vi "Write_CmdMultipleParam.vi"(6 "Command":enum16{"ST"}(ring), 7 "MainParam":i16=-1, 8 "error in (no error)":errorcluster, 9 "Table2":u16[](array[numeric]), 10 "Table1":u16[](array[numeric]), 11 "Multiplexer_Opmux in":refnum<class "Multiplexer_Opmux.lvclass">) -> (0 "error out":errorcluster, 3 "Multiplexer_Opmux out":refnum<class "Multiplexer_Opmux.lvclass">)   [LabVIEW 2014, in "Multiplexer_Opmux.lvclass"]
uses:
  Multiplexer_Opmux.lvclass
  Multiplexer_Opmux.lvclass/Multiplexer_Opmux.ctl
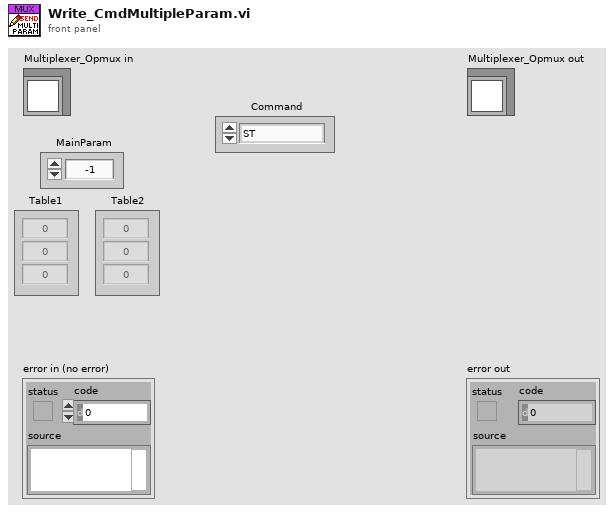
[diagram p1: front panel]
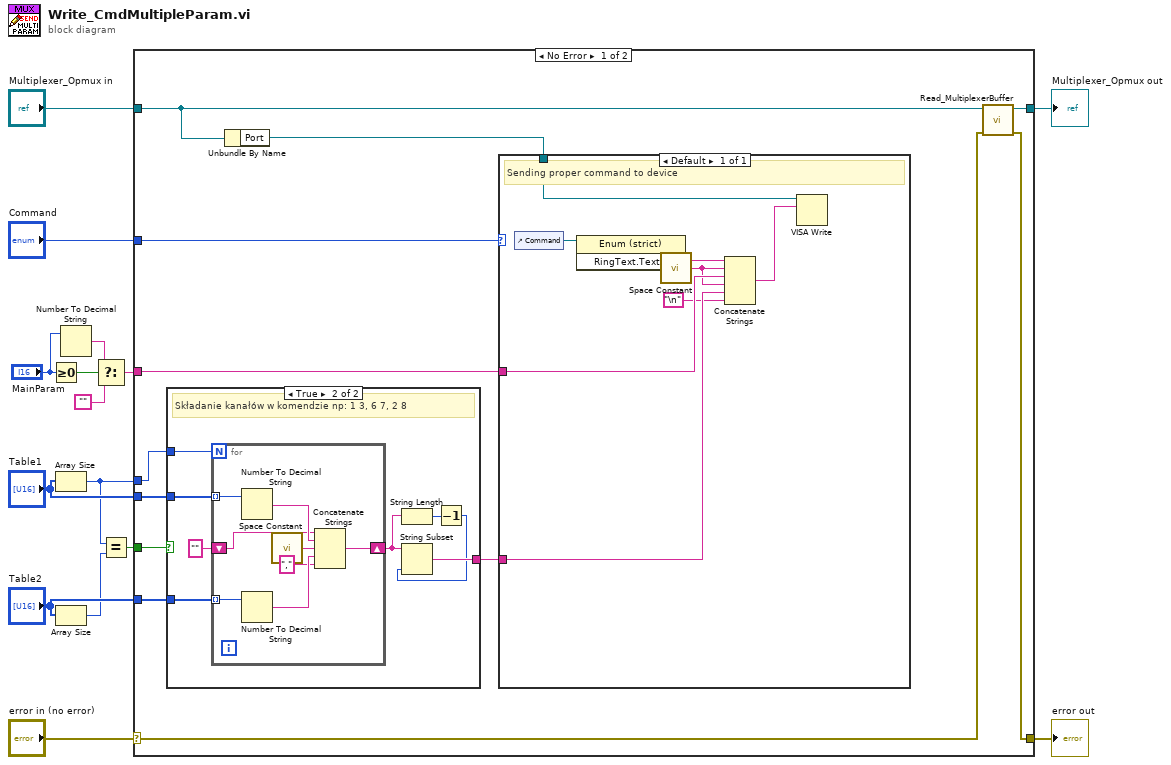
[diagram p0: block diagram]
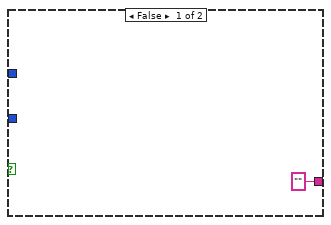
[diagram p2: hidden frame]
diagram:
  n1 = Greater Or Equal To 0?(x="MainParam") -> (x >= 0?=w10:bool)
  n2 = Array Size(array="Table1") -> (size(s)=w1:i32)
  n3 = Array Size(array="Table2") -> (size(s)=w2:i32)
  n4 = Number To Decimal String(number="MainParam") -> (decimal integer string=w9:string)  [unwired: 1 in]
  n5 = Select(t=w9, s=w10, f="") -> (s? t:f=w6:string)
  n6 = Equal?(x=w1, y=w2) -> (x = y?=w4:bool)
  n7 = case shown="No Error" "error in (no error)" {
    selector: "error in (no error)" -> [w17 w54]
    tunnel: [w16 w54] -> w14
    tunnel: [w19 w53] -> w12
    tunnel: "Multiplexer_Opmux in" -> [w18 w53]
    tunnel: "Command" -> [w27 _]
    tunnel: w6 -> [w26 _]
    tunnel: "Table1" -> [w21 _]
    tunnel: w4 -> [w24 _]
    tunnel: "Table2" -> [w22 _]
    tunnel: w1 -> [w23 _]
    frame No Error {
      n8 = case shown="True" w24 {
        tunnel: w23 -> [_ w36]
        tunnel: w22 -> [_ w35]
        tunnel: w21 -> [_ w34]
        tunnel: ["" w31] -> w20
        frame False {
        }
        frame True {
          # "Składanie kanałów w komendzie np: 1 3, 6 7, 2 8"
          n9 = for {
            N: w36 -> [_]
            tunnel: w35 -> [w43] mode=indexing
            tunnel: w34 -> [w44] mode=indexing
            shift-right: [w38] -> w32
            shift-left: "" -> [w37]
            n10 = Number To Decimal String(number=w44) -> (decimal integer string=w42:string)  [unwired: 1 in]
            n11 = Number To Decimal String(number=w43) -> (decimal integer string=w41:string)  [unwired: 1 in]
            n12 = call <vilib>:"Space Constant.vi"() -> ("String"=w40:string)
            n13 = Concatenate Strings(w37, w42, w40, w41, "," ("string")) -> (w38:string)
          }
          n14 = String Length(string=w32) -> (length=w30:i32)
          n15 = Decrement(x=w30) -> (x-1=w29:i32)
          n16 = String Subset(string=w32, length (rest)=w29) -> (substring=w31:string)  [unwired: 1 in]
        }
      }
      n17 = Unbundle By Name(w18) -> ("Port"=w25:refnum<visa-resource-name>)
      n18 = case shown="Default" w27 {
        tunnel: w26 -> [w50]
        tunnel: w25 -> [w46]
        tunnel: w20 -> [w48]
        frame Default {
          # "Sending proper command to device"
          n19 = control-ref of="Command"() -> (w52:refnum<vi>)
          n20 = property class="Enum (strict)"(reference=w52) -> ("RingText.Text"=w51:string)  [unwired: 1 in, 2 out]
          n21 = call <vilib>:"Space Constant.vi"() -> ("String"=w49:string)
          n22 = Concatenate Strings(w51, w49, w50, w49, w48, "\n") -> (w45:string)
          n23 = VISA Write(VISA resource name=w46, write buffer=w45) -> ()  [unwired: 1 in, 3 out]
        }
      }
      n24 = call-dynamic "Read_MultiplexerBuffer.vi"("error in (no error)"=w17, "Multiplexer_Opmux in"=w18) -> ("error out"=w16:errorcluster, "Multiplexer_Opmux out"=w19:refnum<class "Multiplexer_Opmux.lvclass">)  [unwired: 7 in, 1 out]
    }
    frame Error {
    }
  }
  "error out" <- w14
  "Multiplexer_Opmux out" <- w12
